vi "Alarma_IEEE45_G04.vi"(8 "error in (no error)":errorcluster) -> (0 "error out":errorcluster)   [LabVIEW 2018]
uses:
  Controls/Cluster_Alarmas_IEEE45.ctl
  <vilib>/RAFA Solutions/Harmony UI Controls Kit/Boolean/Round Led.ctl
  <vilib>/addons/database/Connection.llb/DB Tools Open Connec (Path).vi
  Global/Demo.vi
  Global/Alarmas_indicadores-LED.vi
  Global/AlarmasGlobal.vi
  <vilib>/addons/database/NI_Database_API.lvlib
  <vilib>/RAFA Solutions/Harmony UI Controls Kit/Flat UI Design.lvlib
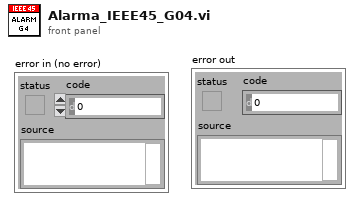
[diagram p1: front panel]
types:
  T1 = typedef "NI_Database_API.lvlib/Conn ObjectReference.ctl" = refnum<k1>
  T2 = typedef "Cluster_Alarmas_IEEE45.ctl" = cluster{"V1_V2 (V) ":cluster{dbl, dbl, dbl}, "Mod_V1_V2":dbl, "alarma 1":T3, "Mod_V2_V3":dbl, "alarma 2":T3, "Mod_V3_V1":dbl, "alarma 3":T3, "Mod_Frec":dbl, "alarma 4":T3, "V2_V3 (V)":cluster{dbl, dbl, dbl}, "V3_V1 (V)":cluster{dbl, dbl, dbl}, "Frecuencia (Hz)":cluster{dbl, dbl, dbl}, "AVG VL_VL (V)":cluster{dbl, dbl, dbl}, "alarm 5":bool, "alarm 6":bool, "alarm 7":bool, "alarm 8":bool, "alarm 9":bool}
  T3 = typedef "Flat UI Design.lvlib/Round Led.ctl" = bool
  T4 = typedef "VIF_cluster.ctl" = cluster{"VL_VL":cluster{"V1_V2":sgl, "V2_V3":sgl, "V3_V1":sgl, "Avg_VL_VL":sgl}, "IL_IL":cluster{"I1":sgl, "I2":sgl, "I3":sgl, "Avg_Amps":sgl}, "Frecuency":sgl, "Avg_Frecuency":sgl}
  T5 = cluster{"V1_V2":sgl, "V2_V3":sgl, "V3_V1":sgl, "Avg_VL_VL":sgl}
  T6 = cluster{"Mod_V1_V2":sgl, "Mod_V2_V3":sgl, "Mod_V3_V1":sgl, "alarma 1":bool, "alarma 2":bool, "alarma 3":bool}
  T7 = cluster{"alarm 5":bool, "alarm 6":bool, "alarm 7":bool, "alarm 8":bool, "alarm 9":bool}
  T8 = cluster{"Frecuency Modulation (%)":sgl, "alarma":bool}
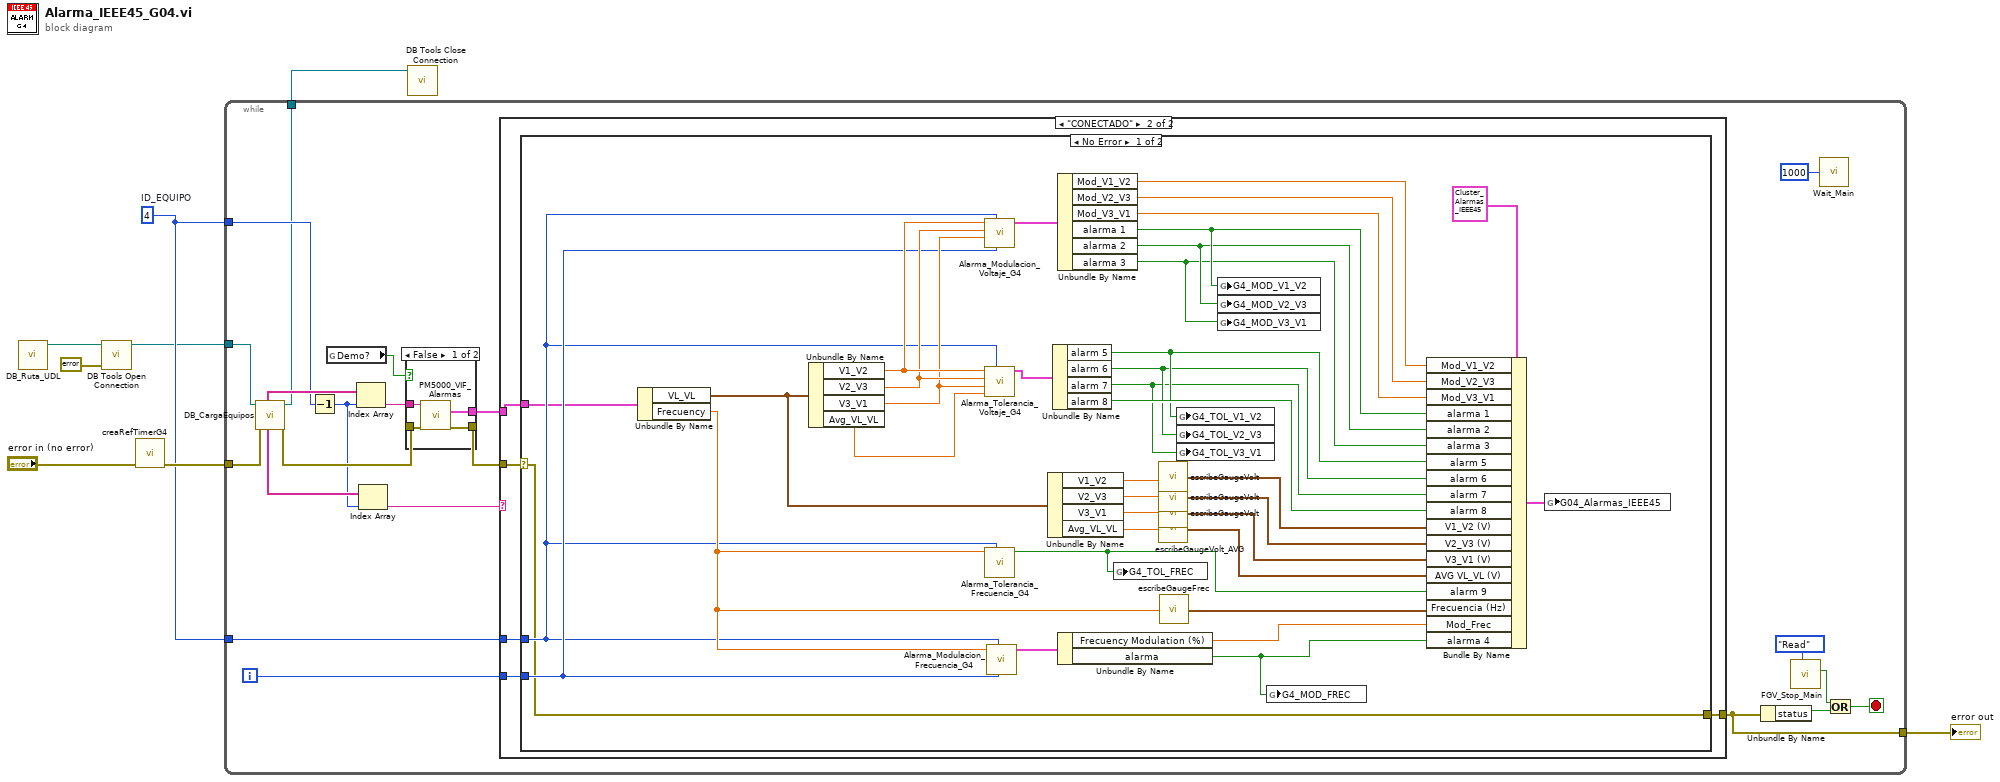
[diagram p0: block diagram]
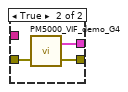
[diagram p2: hidden frame]
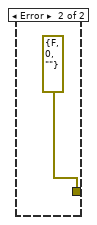
[diagram p4: hidden frame]
diagram:
  w3 = 4  # ID_EQUIPO
  n1 = call "DB_Ruta_UDL.vi"() -> ("UDL ruta"=w4:path)  [unwired: 11 in]
  n2 = call-poly <vilib>:"DB Tools Open Connection.vi"("error in (no error)"=errorcluster {"status"=FALSE, "code"=0, "source"=""}, "connection information"=w4) -> ("connection reference"=w2:T1)  [unwired: 6 in, 1 out]
  n3 = call "creaRefTimerG4.vi"("error in (no error)"="error in (no error)") -> ("error out"=w7:errorcluster)  [unwired: 10 in]
  n4 = while {
    tunnel: w7 -> [w20]
    tunnel: [w23] -> w6
    tunnel: w3 -> [w22]
    tunnel: w3 -> [w19]
    tunnel: w2 -> [w18]
    tunnel: [w17] -> w1
    i -> [w27]
    stop <- w24 stop-if-true
    n5 = call "DB_CargaEquipos.vi"("error in (no error)"=w20, "db in"=w18) -> ("error out"=w15:errorcluster, "db out"=w17:T1, "ESTADO_EQUIPO"=w12:string[], "IP_EQUIPOS"=w21:string[])  [unwired: 2 in, 4 out]
    n6 = Decrement(x=w19) -> (x-1=w11:i32)
    n7 = global read "Demo.vi" "Demo?"() -> (w9:bool)
    n8 = Index Array(array=w21, index=w11) -> (element=w16:string)
    n9 = Index Array(array=w12, index=w11) -> (element=w10:string)
    n10 = case shown="False" w9 {
      tunnel: w16 -> [w33 _]
      tunnel: w15 -> [w32 w36]
      tunnel: [w31 w35] -> w14
      tunnel: [w30 w34] -> w13
      frame False {
        n11 = call "PM5000_VIF_Alarmas.vi"("error in"=w32, "Network Path"=w33) -> ("error out"=w31:errorcluster, "output cluster"=w30:T4)  [unwired: 7 in, 1 out]
      }
      frame True {
        n12 = call "PM5000_VIF_demo_G4.vi"("error in (no error)"=w36) -> ("error out"=w35:errorcluster, "VIF_cluster"=w34:T4)  [unwired: 1 in]
      }
    }
    n13 = case shown="\"CONECTADO\"" w10 {
      tunnel: w27 -> [_ w41]
      tunnel: [_ w40] -> w23
      tunnel: w22 -> [_ w39]
      tunnel: w14 -> [_ w38]
      tunnel: w13 -> [_ w37]
      frame Default {
      }
      frame "CONECTADO" {
        n14 = case shown="No Error" w38 {
          selector: w38 -> [w53 _]
          tunnel: w41 -> [w68 _]
          tunnel: [w53 errorcluster {"status"=FALSE, "code"=0, "source"=""} ("error out")] -> w40
          tunnel: w39 -> [w54 _]
          tunnel: w37 -> [w52 _]
          frame No Error {
            n15 = Unbundle By Name(w52) -> ("VL_VL"=w73:T5, "Frecuency"=w67:sgl)
            n16 = Unbundle By Name(w73) -> ("V1_V2"=w78:sgl, "V2_V3"=w77:sgl, "V3_V1"=w76:sgl, "Avg_VL_VL"=w75:sgl)
            n17 = call "Alarma_Modulacion_Voltaje_G4.vi"("# iteration"=w68, "ID_EQUIPO"=w54, "V3_V1"=w76, "V2_V3"=w77, "V1_V2"=w78) -> ("Alarma_Mod_Volt out"=w74:T6)  [unwired: 6 in]
            n18 = call "Alarma_Tolerancia_Voltaje_G4.vi"("ID_EQUIPO"=w54, "AVG_VL_VL"=w75, "V3_V1"=w76, "V2_V3"=w77, "V1_V2"=w78) -> ("alarm out"=w65:T7)  [unwired: 6 in]
            n19 = call "Alarma_Tolerancia_Frecuencia_G4.vi"("ID_EQUIPO"=w54, "Señal in"=w67) -> ("alarm"=w43:bool)  [unwired: 9 in]
            n20 = call "Alarma_Modulacion_Frecuencia_G4.vi"("# iteration"=w68, "ID_EQUIPO"=w54, "Frecuencia"=w67) -> ("Mod_Frec out"=w66:T8)  [unwired: 8 in]
            n21 = Unbundle By Name(w73) -> ("V1_V2"=w72:sgl, "V2_V3"=w71:sgl, "V3_V1"=w70:sgl, "Avg_VL_VL"=w69:sgl)
            n22 = Unbundle By Name(w65) -> ("alarm 5"=w46:bool, "alarm 6"=w45:bool, "alarm 7"=w44:bool, "alarm 8"=w61:bool)
            n23 = Unbundle By Name(w74) -> ("Mod_V1_V2"=w64:sgl, "Mod_V2_V3"=w63:sgl, "Mod_V3_V1"=w62:sgl, "alarma 1"=w49:bool, "alarma 2"=w48:bool, "alarma 3"=w47:bool)
            n24 = Unbundle By Name(w66) -> ("Frecuency Modulation (%)"=w55:sgl, "alarma"=w42:bool)
            n25 = global write "Alarmas_indicadores-LED.vi" "G4_TOL_FREC"(w43) -> ()
            n26 = call "escribeGaugeVolt.vi"("Vin"=w72) -> ("V_V out"=w60:cluster{"Max":sgl, "Vin":sgl, "Min":sgl})
            n27 = call "escribeGaugeVolt.vi"("Vin"=w71) -> ("V_V out"=w59:cluster{"Max":sgl, "Vin":sgl, "Min":sgl})
            n28 = call "escribeGaugeVolt.vi"("Vin"=w70) -> ("V_V out"=w58:cluster{"Max":sgl, "Vin":sgl, "Min":sgl})
            n29 = call "escribeGaugeVolt_AVG.vi"("Vin"=w69) -> ("V_V out"=w57:cluster{"Max":sgl, "Vin":sgl, "Min":sgl})
            n30 = call "escribeGaugeFrec.vi"("Fin"=w67) -> ("Frec out"=w56:cluster{"Max":sgl, "Vin":sgl, "Min":sgl})
            n31 = global write "Alarmas_indicadores-LED.vi" "G4_TOL_V1_V2"(w46) -> ()
            n32 = global write "Alarmas_indicadores-LED.vi" "G4_TOL_V2_V3"(w45) -> ()
            n33 = global write "Alarmas_indicadores-LED.vi" "G4_TOL_V3_V1"(w44) -> ()
            n34 = global write "Alarmas_indicadores-LED.vi" "G4_MOD_V1_V2"(w49) -> ()
            n35 = global write "Alarmas_indicadores-LED.vi" "G4_MOD_V2_V3"(w48) -> ()
            n36 = global write "Alarmas_indicadores-LED.vi" "G4_MOD_V3_V1"(w47) -> ()
            n37 = global write "Alarmas_indicadores-LED.vi" "G4_MOD_FREC"(w42) -> ()
            n38 = Bundle By Name(cluster=T2 {"V1_V2 (V) "={0.0, 17.0, 16.662651515468255}, "Mod_V1_V2"=0.0, "alarma 1"=FALSE, "Mod_V2_V3"=0.0, "alarma 2"=FALSE, "Mod_V3_V1"=0.0, "alarma 3"=FALSE, "Mod_Frec"=0.0, "alarma 4"=FALSE, "V2_V3 (V)"={0.0, 17.0, 16.662651515468255}, "V3_V1 (V)"={0.0, 17.0, 16.662651515468255}, "Frecuencia (Hz)"={0.0, 17.0, 16.662651515468255}, "AVG VL_VL (V)"={0.0, 17.0, 16.662651515468255}, "alarm 5"=FALSE, "alarm 6"=FALSE, "alarm 7"=FALSE, "alarm 8"=FALSE, "alarm 9"=FALSE} ("G04_Alarmas_IEEE45"), "Mod_V1_V2"=w64, "Mod_V2_V3"=w63, "Mod_V3_V1"=w62, "alarma 1"=w49, "alarma 2"=w48, "alarma 3"=w47, "alarm 5"=w46, "alarm 6"=w45, "alarm 7"=w44, "alarm 8"=w61, "V1_V2 (V)"=w60, "V2_V3 (V)"=w59, "V3_V1 (V)"=w58, "AVG VL_VL (V)"=w57, "alarm 9"=w43, "Frecuencia (Hz)"=w56, "Mod_Frec"=w55, "alarma 4"=w42) -> (w50:T2)
            n39 = global write "AlarmasGlobal.vi" "G04_Alarmas_IEEE45"(w50) -> ()
          }
          frame Error {
          }
        }
      }
    }
    n40 = Unbundle By Name(w23) -> ("status"=w25:bool)
    n41 = call "FGV_Stop_Main.vi"("Action"=enum16{"Read", "Write"}."Read") -> ("Var Out"=w26:bool)  [unwired: 9 in, 1 out]
    n42 = call "Wait_Main.vi"("Wait time (msec)"=u32 1000 ("delay (ms)")) -> ()  [unwired: 5 in]
    n43 = Or(x=w26, y=w25) -> (x .or. y?=w24:bool)
  }
  "error out" <- w6
  n44 = call <vilib>:"DB Tools Close Connection.vi"("connection reference"=w1) -> ()  [unwired: 6 in, 1 out]
